vi "Connection Engine.vi"(8 "error in (no error)":errorcluster, 11 "State Variables":T1) -> (0 "error out":errorcluster)   [LabVIEW 2015, in "Instrument Addon Engine.lvlib" / "Network Common API.lvlib"]
uses:
  Network Common API.lvlib
  Inline Async API/Controls/Engine State Variables.ctl
  TCP Refs.ctl
  Network Comm Global Ref.ctl
  Stop FG/Stop Global Ref.ctl
  <vilib>/NI/AMC/Message Queue.ctl
  <vilib>/NI/AMC/Message.ctl
  <vilib>/NI/Tools/Keyed Array/KeyedArray.ctl
  Stop FG/Stop Global Commands.ctl
  <userlib>/STM/TCP/stm_TCP Read Options.ctl
  <userlib>/STM/Connection Manager/TCP/stm_TCPConnectionMethod.ctl
  <userlib>/STM/Connection Manager/TCP/stm_TCPConnectionProperties.ctl
  <userlib>/STM/TCP/STM Get Connection Reference (TCP).vi
  <userlib>/STM/TCP/STM Read Meta Data (TCP Ref).vi
  <vilib>/NI Veristand/Custom Device Tools/Custom Device Utility Library/Custom Device Utility Library.lvlib
  Stop FG/Stop FG.lvlib
  Error Handling API/Error Handling API.lvlib
  Inline Async API/Inline Async API.lvlib
  <vilib>/NI/Tools/Keyed Array/Tools_KeyedArray.lvlib
  <vilib>/NI/AMC/AMC.lvlib
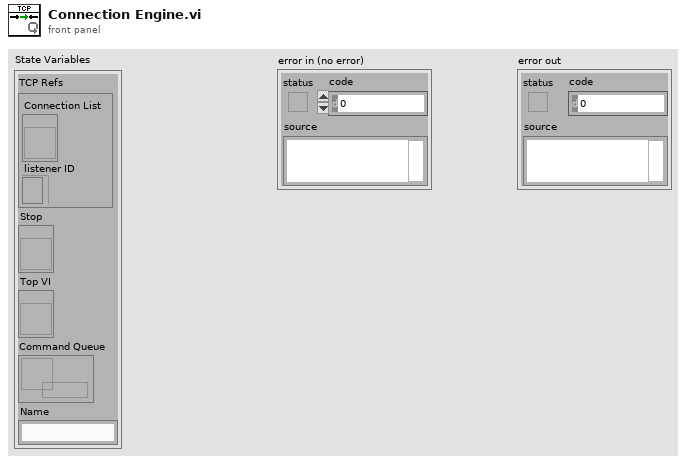
[diagram p1: front panel]
types:
  T1 = typedef "Instrument Addon Engine.lvlib/Inline Async API.lvlib/Engine State Variables.ctl" = cluster{"TCP Refs":T2, "Stop":T4, "Top VI":refnum<vi>, "Command Queue":T5, "Name":string}
  T2 = typedef "Instrument Addon Engine.lvlib/Network Common API.lvlib/TCP Refs.ctl" = cluster{"Connection List":T3, "listener ID":refnum<k5>}
  T3 = typedef "Instrument Addon Engine.lvlib/Network Common API.lvlib/Network Comm Global Ref.ctl" = refnum<vi>
  T4 = typedef "Instrument Addon Engine.lvlib/Stop FG.lvlib/Stop Global Ref.ctl" = refnum<vi>
  T5 = typedef "AMC.lvlib/Message Queue.ctl" = refnum<queue>
  T6 = typedef "Instrument Addon Engine.lvlib/Stop FG.lvlib/Stop Global Commands.ctl" = enum16{"Write", "Read", "Reset"}
  T7 = typedef "stm_TCP Read Options.ctl" = cluster{"Ignore Timeout Error":bool, "timeout ms (1000)":i32}
  T8 = typedef "stm_TCPConnectionProperties.ctl" = cluster{"Name":string, "Address":string, "Custom":string}
  T9 = typedef "stm_TCPConnectionMethod.ctl" = enum16{"Initialize", "Add Connection", "Set Properties", "Get Connection(s)", "Remove Connection", "Remove All Connections", "Get Connection Count"}
  T10 = typedef "stm_TCP Connection Info.ctl" = cluster{"connection ID":refnum<k5>, "Meta data":T11[]}
  T11 = typedef "stm_MetaDataElement.ctl" = string
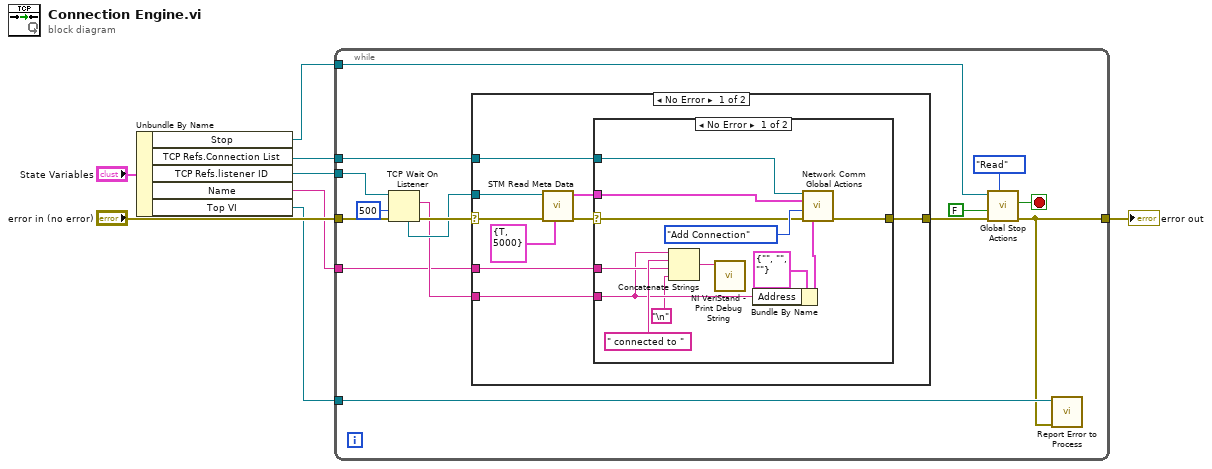
[diagram p0: block diagram]
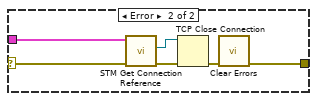
[diagram p2: hidden frame]
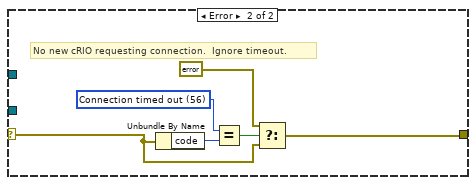
[diagram p3: hidden frame]
diagram:
  n1 = Unbundle By Name("State Variables") -> ("Stop"=w8:T4, "TCP Refs.Connection List"=w6:T3, "TCP Refs.listener ID"=w7:refnum<k5>, "Name"=w1:string, "Top VI"=w2:refnum<vi>)
  n2 = while {
    tunnel: "error in (no error)" -> [w23]
    tunnel: w7 -> [w22]
    tunnel: w8 -> [w15]
    tunnel: [w9] -> w3
    tunnel: w6 -> [w13]
    tunnel: w1 -> [w12]
    tunnel: w2 -> [w10]
    stop <- w17 stop-if-true
    n3 = TCP Wait On Listener(8:w23, 9:500 ("timeout ms (wait forever: -1)"), 11:w22) -> (0:w20:errorcluster, 2:w18:string, 4:w19:refnum<k5>)  [unwired: 1 in, 2 out]
    n4 = case shown="No Error" w20 {
      selector: w20 -> [w32 w52]
      tunnel: w19 -> [w27 _]
      tunnel: [w31 w53] -> w16
      tunnel: w18 -> [w29 _]
      tunnel: w13 -> [w30 _]
      tunnel: w12 -> [w28 _]
      frame No Error {
        n5 = call-poly <userlib>:"STM Read Meta Data.vi"("Options"=T7 {"Ignore Timeout Error"=TRUE, "timeout ms (1000)"=5000} ("options"), "error in"=w32, "connection ID"=w27) -> ("error out"=w26:errorcluster, "Connection Info Out"=w25:T10)  [unwired: 6 in, 1 out]
        n6 = case shown="No Error" w26 {
          selector: w26 -> [w40 w47]
          tunnel: w30 -> [w38 _]
          tunnel: w25 -> [w39 w48]
          tunnel: [w41 w50] -> w31
          tunnel: w29 -> [w34 _]
          tunnel: w28 -> [w35 _]
          frame No Error {
            n7 = Concatenate Strings(w34, " connected to " ("string"), w35, "\n") -> (w36:string)
            n8 = call <vilib>:"NI VeriStand - Print Debug String.vi"("Message"=w36) -> ()  [unwired: 10 in, 1 out]
            n9 = Bundle By Name(cluster=T8 {"Name"="", "Address"="", "Custom"=""} ("Properties In"), "Address"=w34) -> (w44:T8)
            n10 = call "Network Comm Global Actions.vi"("ref in"=w38, "Connection In"=w39, "Method"=stm_TCPConnectionMethod."Add Connection", "error in (no error)"=w40, "Properties In"=w44) -> ("error out"=w41:errorcluster)  [unwired: 4 in, 6 out]
          }
          frame Error {
            n11 = call-poly <userlib>:"STM Get Connection Reference.vi"("error in"=w47, "Connection Info"=w48) -> ("error out"=w45:errorcluster, "connection ID out"=w46:refnum<k5>)  [unwired: 7 in, 1 out]
            n12 = TCP Close Connection(connection ID=w46, error in (no error)=w45) -> (error out=w49:errorcluster)  [unwired: 1 in, 1 out]
            n13 = call <vilib>:"Clear Errors.vi"("error in (no error)"=w49) -> ("error out"=w50:errorcluster)  [unwired: 5 in, 1 out]
          }
        }
      }
      frame Error {
        w51 = 56 items=["No Error", "Argument Error", "Memory Full", "Out of Zone", "End of File", "File Already Open", "Generic File IO Error", "File Not Found", "File Permission Error", "Disk Full", "Duplicate Path", "Too Many Files Open", "Not Enabled", "Resource File Not Found", "Cannot Add Resource", "Resource Not Found", "Image Not Found", "Image Memory Error", "Pen Does Not Exist", "Config Bad Type", "Config Token Not Found", "Config Parse Error", "Config Memory Error", "Bad External Code Format", "Bad External Code Offset", "External Code Not Present", "Null Window", "Destroy Window Mixup", "Null Menu", "Print Aborted", "Bad Print Record", "Print Driver Error", "Windows Error During Print", "Memory Error During Print", "Print Dialog Error", "Generic Print Error", "Invalid Device Refnum", "Device Not Found", "Device Parameter Error", "Device Unit Error", "Can't Open Device", "Device Call Aborted", "Generic Error", "Cancelled By User", "Object ID Too Low", "Object ID Too High", "Object Not In Heap", "Unknown Heap", "Bad DefProc ID", "DefProc Not In Table", "Message Out Of Range", "Null Method", "Unknown Message", "Manager Call Not Supported", "Bad address", "Connection In progress", "Connection timed out", "Connection is already in progress", "Network attribute not supported", "Network error", "Address in use", "System out of memory", "Connection aborted", "Connection refused", "Connection is not connected", "Connection is already connected", "Connection closed", "Initialize error (interapplication manager)", "Bad occurrence", "Wait on unbound occurrence handler", "Occurrence queue overflow", "Bad path", "Semaphore not signaled", "Unrecognized type (interapplication manager)"] ("1st Error to Convert")
        # "No new cRIO requesting connection.  Ignore timeout."
        n14 = Unbundle By Name(w52) -> ("code"=w55:i32)
        n15 = Equal?(x=w51, y=w55) -> (x = y?=w56:bool)
        n16 = Select(t=errorcluster {"status"=FALSE, "code"=0, "source"=""} ("error in (no error)"), s=w56, f=w52) -> (s? t:f=w53:errorcluster)
      }
    }
    n17 = call "Global Stop Actions.vi"("Command"=Stop_Global_Commands."Read", "error in (no error)"=w16, "Stop on Error?"=FALSE, "vi reference"=w15) -> ("error out"=w9:errorcluster, "Latched Stop"=w17:bool)  [unwired: 5 in, 1 out]
    n18 = call "Report Error to Process.vi"("Error"=w9, "This VI"=w10) -> ()  [unwired: 10 in]
  }
  "error out" <- w3
